vi "SharedHeader.vi"(1 "Write?":bool, 2 "HeaderInput":string) -> (0 "Header":string)   [LabVIEW 2010, in "Player.lvlib"]
uses:
  Player.lvlib
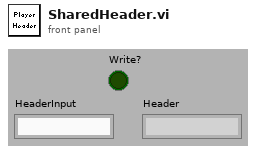
[diagram p1: front panel]
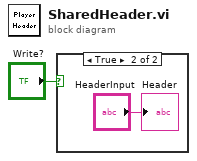
[diagram p0: block diagram]
diagram:
  n1 = case shown="True" "Write?" {
    frame False {
    }
    frame True {
      "Header" <- "HeaderInput"
    }
  }
